vi "Launch Step Trigger VI.vi"(8 "error in (no error)":errorcluster, 11 "Device Item Ref in":T1=18446744073709551615 format="%.0x") -> (0 "error out":errorcluster)   [LabVIEW 2019, in "TimingDRV System Explorer.lvlib"]
uses:
  TimingDRV System Explorer.lvlib
  <vilib>/NI VeriStand/Custom Device API/Custom Device Item Ref.ctl
  <vilib>/NI VeriStand/Custom Device API/Custom Device API.lvlib
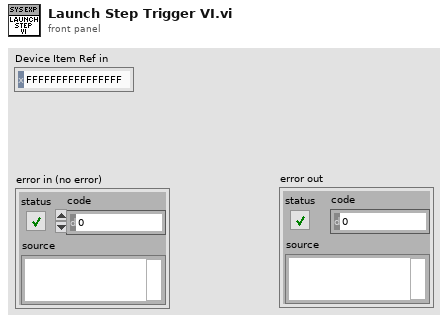
[diagram p1: front panel]
types:
  T1 = typedef "Custom Device API.lvlib/Custom Device Item Ref.ctl" = u64
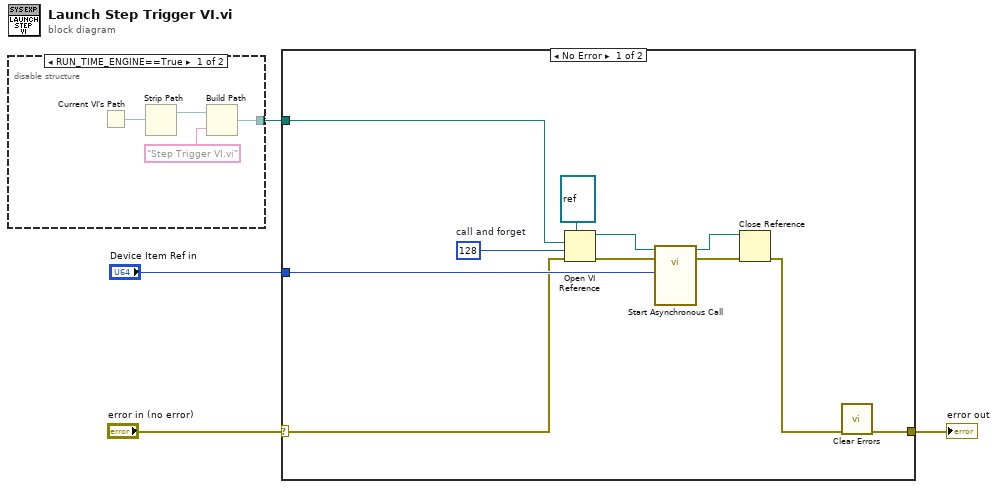
[diagram p0: block diagram]
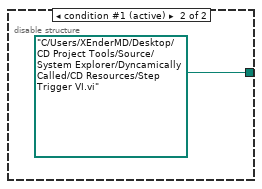
[diagram p3: hidden frame]
diagram:
  n1 = disable-structure shown="RUN_TIME_ENGINE==True" {
    disable-tunnel: [w5 path "C:/Users/XEnderMD/Desktop/CD Project Tools/Source/System Explorer/Dyncamically Called/CD Resources/Step Trigger VI.vi" ("appended path")] -> w3
    frame condition #0 {
      n2 = Current VI's Path() -> (path=w8:path)
      n3 = Strip Path(path=w8) -> (stripped path=w7:path)  [unwired: 1 out]
      n4 = Build Path(base path=w7, name or relative path="Step Trigger VI.vi") -> (appended path=w5:path)
    }
    frame condition #1 (active) {
    }
  }
  n5 = case shown="No Error" "error in (no error)" {
    selector: "error in (no error)" -> [w10 w21]
    tunnel: [w19 w21] -> w4
    tunnel: w3 -> [w20 _]
    tunnel: "Device Item Ref in" -> [w11 _]
    frame No Error {
      w17 = 128  # call and forget
      n6 = Open VI Reference(type specifier VI Refnum (for type only)=refnum<vi> refnum, vi path=w20, options=w17, error in (no error)=w10) -> (vi reference=w14:refnum<vi>, error out=w15:errorcluster)  [unwired: 2 in]
      n7 = call-by-ref "Start Asynchronous Call"(reference=w14, error in=w15, "Device Item Ref in"=w11) -> (reference out=w12:refnum<vi>, error out=w13:errorcluster)  [unwired: 9 in, 2 out]
      n8 = Close Reference(reference=w12, error in (no error)=w13) -> (error out=w18:errorcluster)
      n9 = call <vilib>:"Clear Errors.vi"("error in (no error)"=w18) -> ("error out"=w19:errorcluster)  [unwired: 5 in, 1 out]
    }
    frame Error {
    }
  }
  "error out" <- w4
